vi "Voltage to Pressure.vi"(8 "x":dbl[](array[numeric]), 10 "Vmax":dbl, 11 "Pmax":dbl) -> (3 "pressureOut":dbl[](array[numeric]))   [LabVIEW 2021, in "Interface-Module.lvlib"]
uses:
  Interface-Module/Interface-Module.lvlib
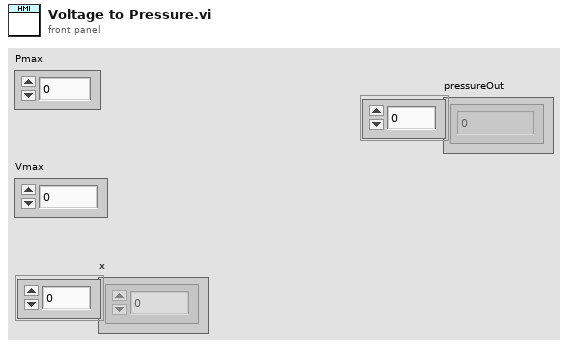
[diagram p1: front panel]
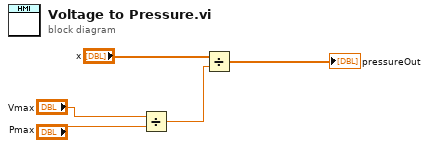
[diagram p0: block diagram]
diagram:
  n1 = Divide(x="Vmax", y="Pmax") -> (x/y=w2:dbl)
  n2 = Divide(x="x", y=w2) -> (x/y=→"pressureOut":dbl[])
